vi "GetParam.vi"(8 "error in (no error)":errorcluster caption="entrée d'erreur (pas d'erreur)", 11 "Sparse_Spd_Matrix.lvclass":refnum<class "Sparse_Spd_Matrix.lvclass">) -> (0 "error out":errorcluster caption="sortie d'erreur", 2 "make_sparse_spd_matrix":T1={"dim"=1, "alpha"=0.95, "norm_diag"=FALSE, " smallest_coef"=0.1, "largest_coef"=0.9, "random_state"=-1} {"random_state" min=-1; "largest_coef" min=0.0 max=1.0; "smallest_coef" min=0.0 max=1.0; "alpha" min=0.0 max=1.0; "dim" min=1}, 3 "Sparse_Spd_Matrix.lvclass":refnum<class "Sparse_Spd_Matrix.lvclass">)   [LabVIEW 2020, in "Sparse_Spd_Matrix.lvclass"]
doc: "Get Parameters"
uses:
  Sparse_Spd_Matrix.lvclass
  Sparse_Spd_Matrix.lvclass/Sparse_Spd_Matrix.ctl
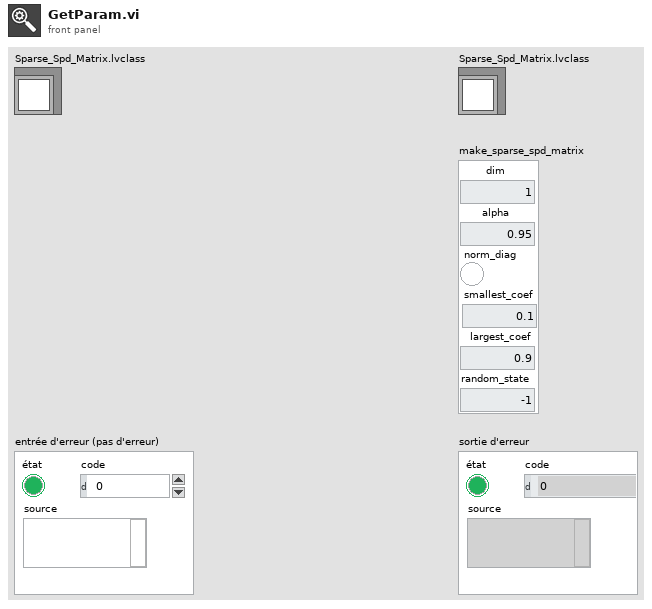
[diagram p1: front panel]
types:
  T1 = cluster{"dim":u32, "alpha":dbl, "norm_diag":bool, " smallest_coef":dbl, "largest_coef":dbl, "random_state":i32}
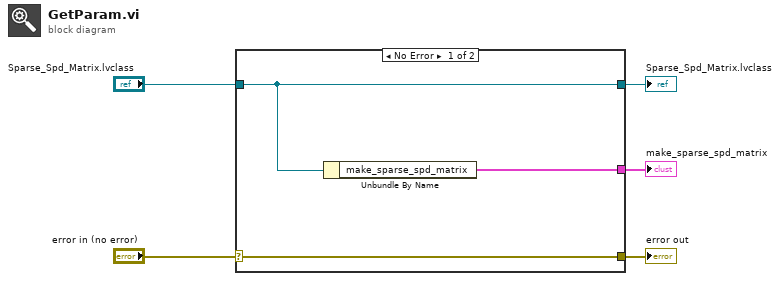
[diagram p0: block diagram]
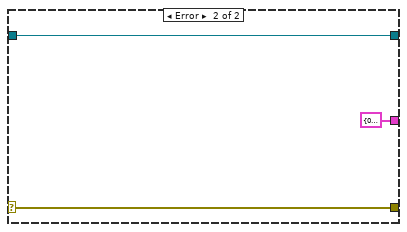
[diagram p2: hidden frame]
diagram:
  n1 = case shown="No Error" "error in (no error)" {
    selector: "error in (no error)" -> [w8 w10]
    tunnel: [w8 w10] -> w4
    tunnel: [w7 w11] -> w2
    tunnel: "Sparse_Spd_Matrix.lvclass" -> [w7 w11]
    tunnel: [w6 T1 {"dim"=0, "alpha"=0.0, "norm_diag"=FALSE, " smallest_coef"=0.0, "largest_coef"=0.0, "random_state"=0} ("make_sparse_spd_matrix")] -> w1
    frame No Error {
      n2 = Unbundle By Name(w7) -> ("make_sparse_spd_matrix"=w6:T1)
    }
    frame Error {
    }
  }
  "error out" <- w4
  "Sparse_Spd_Matrix.lvclass" <- w2
  "make_sparse_spd_matrix" <- w1
